vi "DCPower_CreateOutputArray_V3.vi"(4 "current measurements":dbl[](array[numeric]), 6 "voltage measurements":dbl[](array[numeric]), 7 "Time Stamp Array":timestamp, 8 "error in":errorcluster, 9 "actual count":i32, 10 "Measure Record dt":dbl, 11 "Initial Time":timestamp) -> (0 "error out":errorcluster, 3 "Data Output Array":dbl[][](array[numeric]))   [LabVIEW 2019]
uses:
  <vilib>/Analysis/1siggen.llb/Ramp Pattern by Delta.vi
  <vilib>/Analysis/NI_AALBase.lvlib
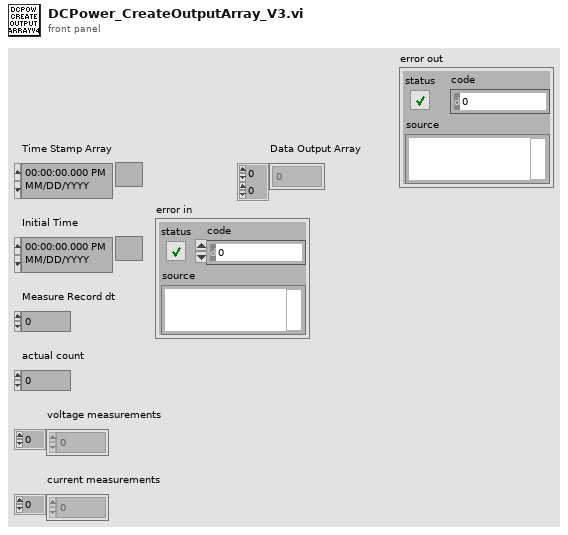
[diagram p1: front panel]
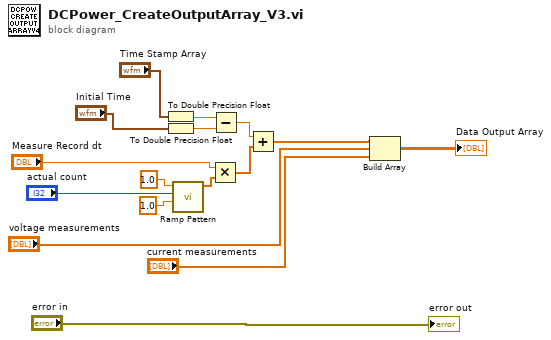
[diagram p0: block diagram]
diagram:
  n1 = To Double Precision Float(number="Time Stamp Array") -> (double precision float=w4:dbl)
  n2 = To Double Precision Float(number="Initial Time") -> (double precision float=w5:dbl)
  n3 = call-poly <vilib>:"Ramp Pattern.vi"("start"=1.0, "end"="actual count", "delta"=1.0) -> ("Ramp Pattern"=w8:dbl[])  [unwired: 6 in, 2 out]
  n4 = Multiply(x="Measure Record dt", y=w8) -> (x*y=w9:dbl[])
  n5 = Subtract(x=w4, y=w5) -> (x-y=w7:dbl)
  n6 = Add(x=w7, y=w9) -> (x+y=w2:dbl[])
  n7 = Build Array(w2, "voltage measurements", "current measurements") -> (→"Data Output Array":dbl[][])
  "error out" <- "error in"
